vi "slope_calculation.vi"(1 "Solar azimuth angle (rad)":dbl, 2 "Slope azimuth angle (rad)":dbl, 3 "Slope angle (rad)":dbl, 4 "Zenith angle (rad)":dbl) -> (0 "cos theta hat / cos Z":dbl)   [LabVIEW 2012]
panel:
  out "cos theta":dbl
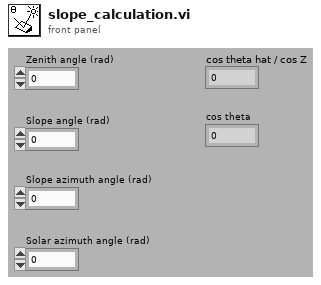
[diagram p1: front panel]
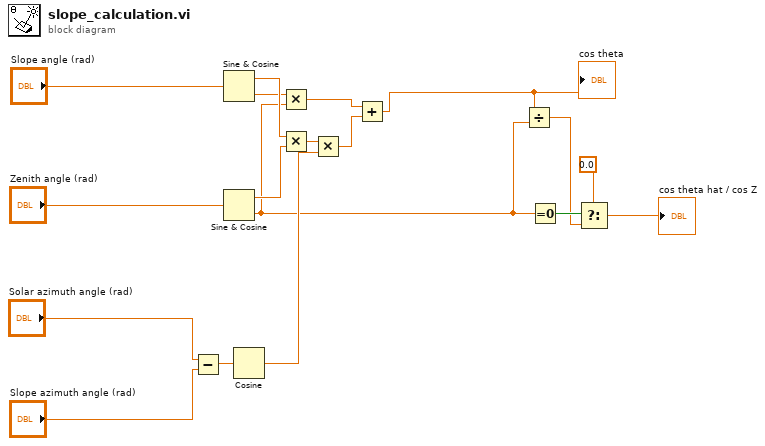
[diagram p0: block diagram]
diagram:
  n1 = Subtract(x="Solar azimuth angle (rad)", y="Slope azimuth angle (rad)") -> (x-y=w13:dbl)
  n2 = Sine & Cosine(0:"Slope angle (rad)") -> (1:w9:dbl, 2:w7:dbl)
  n3 = Sine & Cosine(0:"Zenith angle (rad)") -> (1:w8:dbl, 2:w6:dbl)
  n4 = Cosine(x=w13) -> (cos(x)=w12:dbl)
  n5 = Multiply(x=w7, y=w6) -> (x*y=w18:dbl)
  n6 = Multiply(x=w9, y=w8) -> (x*y=w17:dbl)
  n7 = Multiply(x=w17, y=w12) -> (x*y=w16:dbl)
  n8 = Add(x=w18, y=w16) -> (x+y=w1:dbl)
  "cos theta" <- w1
  n9 = Divide(x=w1, y=w6) -> (x/y=w4:dbl)
  n10 = Equal To 0?(x=w6) -> (x = 0?=w5:bool)
  n11 = Select(t=0.0, s=w5, f=w4) -> (s? t:f=→"cos theta hat / cos Z":dbl)
